vi "file list -- accumulate V2.vi"(11 "file path":path=path "/snowfall/Users/arcadi/Desktop/Ultrasound/Experiment/YBCO_4/Round1/Sweep12/June_2011/062511/221.16400K_300_3100_001_062511.dat") -> (0 "timestamp":dbl[](array[numeric]), 2 "sweep file name array":T1[](array[typedef]), 3 "temperatures":dbl[](array[numeric]))   [LabVIEW 2010]
uses:
  sweep file name.ctl
  <vilib>/Utility/file.llb/Read From Spreadsheet File (string).vi
panel:
  in  "dummy 2":T1={"temperature"=0.0, "temperature str"="", "file path"=path "/snowfall/Users/arcadi/Desktop/Ultrasound/Experiment/YBCO_4/Round1/Sweep12/June_2011/062511/221.16400K_300_3100_001_062511.dat", "last mod"=timestamp(0 s since 1904-01-01), "file name str"="", "mod time(min)"=0.0, "file format"=enum.""}
  in  "sweep file name":T1={"temperature"=0.0, "temperature str"="", "file path"=path "/snowfall/Users/arcadi/Desktop/Ultrasound/Experiment/YBCO_4/Round1/Sweep12/June_2011/062511/221.16400K_300_3100_001_062511.dat", "last mod"=timestamp(0 s since 1904-01-01), "file name str"="", "mod time(min)"=0.0, "file format"=enum.""}
  in  "dummy":T1={"temperature"=0.0, "temperature str"="", "file path"=path "/snowfall/Users/arcadi/Desktop/Ultrasound/Experiment/YBCO_4/Round1/Sweep12/June_2011/062511/221.16400K_300_3100_001_062511.dat", "last mod"=timestamp(0 s since 1904-01-01), "file name str"="", "mod time(min)"=0.0, "file format"=enum.""}
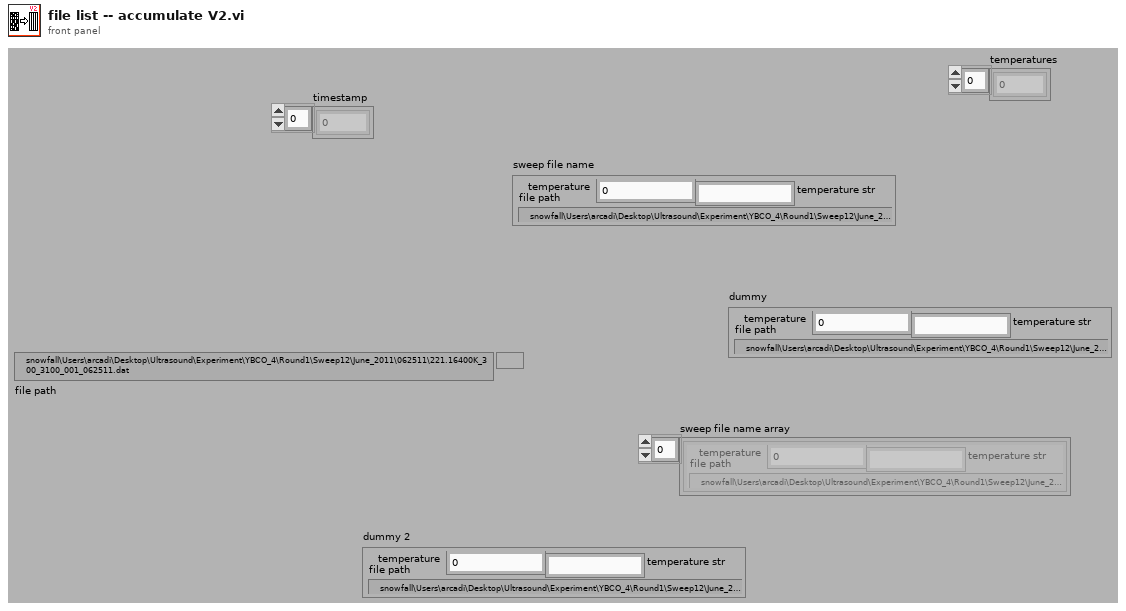
[diagram p1: front panel]
types:
  T1 = typedef "sweep file name.ctl" = cluster{"temperature":dbl, "temperature str":string, "file path":path, "last mod":timestamp, "file name str":string, "mod time(min)":dbl, "file format":enum16{"", "ascii", "binary"}}
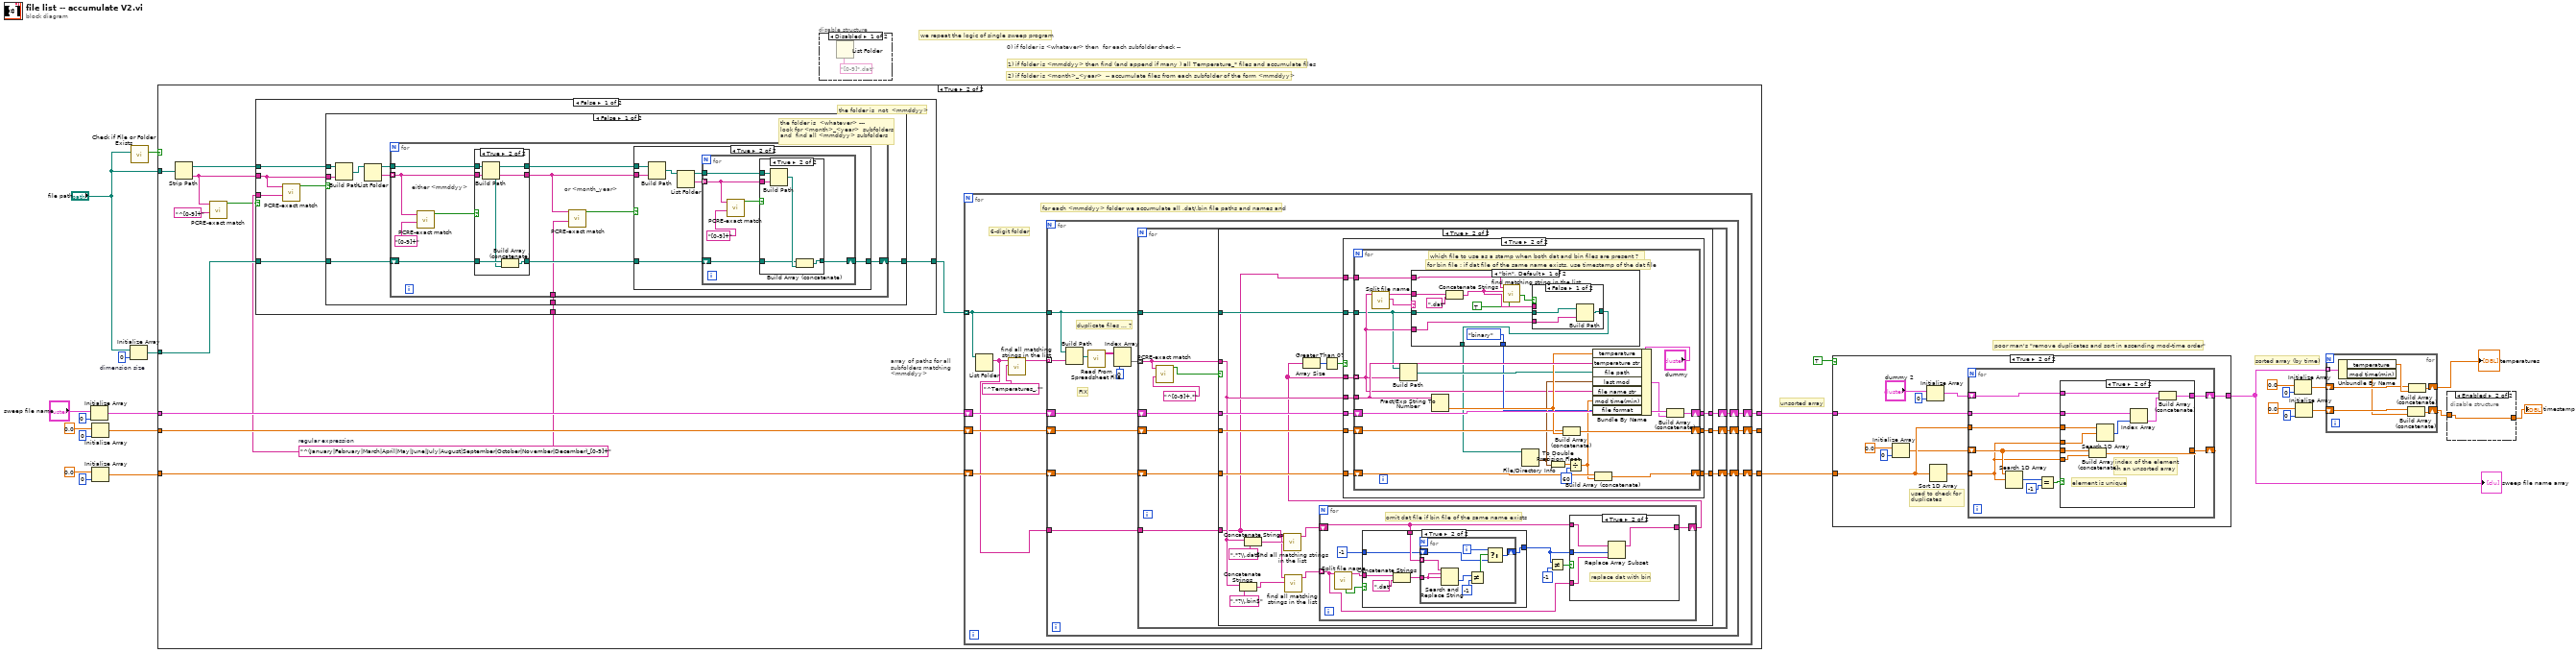
[diagram p0: block diagram]
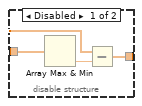
[diagram p2: hidden frame]
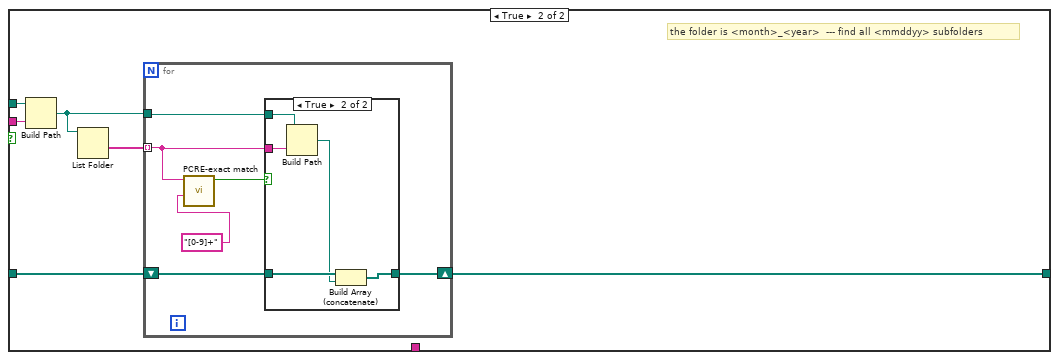
[diagram p10: hidden frame]
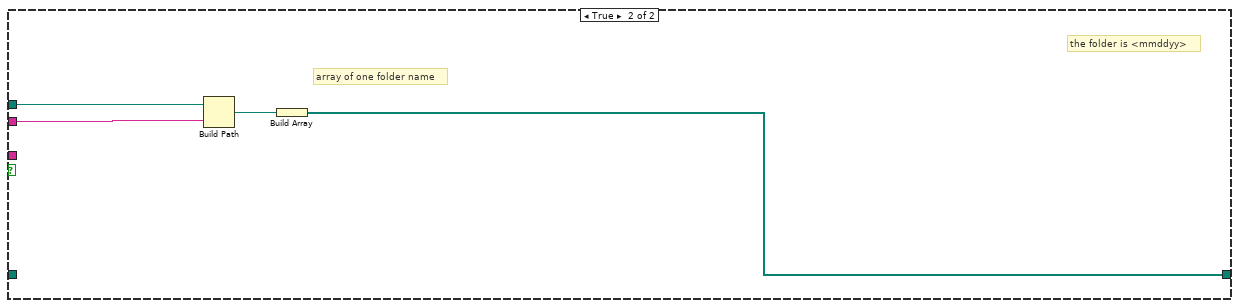
[diagram p12: hidden frame]
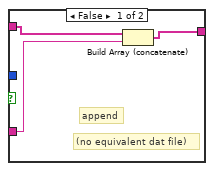
[diagram p14: hidden frame]
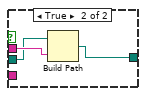
[diagram p17: hidden frame]
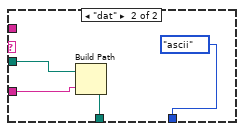
[diagram p18: hidden frame]
diagram:
  w3 = 0  # dimension size
  # "0) if folder is <whatever> then  for each subfolder check --"
  # "sorted array (by time)"
  # "unsorted array"
  # "poor man's \"remove duplicates and sort in ascending mod-time order\""
  # "1) if folder is <mmddyy> then find (and append if many ) all Temperature_* files and accumulate files"
  # "2) if folder is <month>_<year>  -- accumulate files from each subfolder of the form <mmddyy>"
  # "we repeat the logic of single sweep program"
  n1 = Initialize Array("sweep file name", 0 ("dimension size")) -> (w21:T1[])
  n2 = Initialize Array(0.0 ("dimension size"), 0 ("dimension size")) -> (w20:dbl[])
  n3 = Initialize Array(0.0 ("dimension size"), 0 ("dimension size")) -> (w17:dbl[])
  n4 = Initialize Array("file path", w3) -> (w1:path[])
  n5 = call <vilib>:"Check if File or Folder Exists.vi"("path"="file path") -> ("file or folder exists?"=w26:bool)  [unwired: 8 in, 2 out]
  n6 = case shown="True" w26 {
    tunnel: "file path" -> [_ w39]
    tunnel: [w29 w41] -> w14
    tunnel: [w28 w40] -> _
    tunnel: w21 -> [w29 w43]
    tunnel: w20 -> [w28 w42]
    tunnel: w17 -> [w27 w38]
    tunnel: [w27 w37] -> w15
    tunnel: w1 -> [_ w34]
    frame False {
    }
    frame True {
      w33 = "^(January|February|March|April|May|June|July|August|September|October|November|December)_[0-9]+"  # regular expression
      # "array of paths for all  \nsubfolders matching\n<mmddyy>"
      n7 = Strip Path(path=w39) -> (stripped path=w36:path, name=w32:string)
      n8 = call "PCRE-exact match.vi"("regular expression"="^[0-9]+", "input string"=w32) -> ("exact match"=w30:bool)  [unwired: 8 in, 1 out]
      n9 = case shown="False" w30 {
        tunnel: [w50 w118] -> w35
        tunnel: w36 -> [w49 w117]
        tunnel: w32 -> [w45 w116]
        tunnel: w33 -> [w46 _]
        tunnel: w34 -> [w48 _]
        tunnel: w33 -> [w47 _]
        frame False {
          # "the folder is  not  <mmddyy>"
          n10 = call "PCRE-exact match.vi"("regular expression"=w46, "input string"=w45) -> ("exact match"=w44:bool)  [unwired: 8 in, 1 out]
          n11 = case shown="False" w44 {
            tunnel: [w52 w101] -> w50
            tunnel: w45 -> [w55 w100]
            tunnel: w49 -> [w56 w99]
            tunnel: w48 -> [w54 w98]
            tunnel: w47 -> [w53 _]
            frame False {
              # "the folder is  <whatever> --- \nlook for <month>_<year>  subfolders \nand  find all <mmddyy> subfolders"
              n12 = Build Path(base path=w56, name or relative path=w55) -> (appended path=w57:path)
              n13 = List Folder(path=w57) -> (path out=w51:path, folder names=w58:string[])  [unwired: 3 in, 2 out]
              n14 = for {
                tunnel: w58 -> [w64] mode=indexing
                shift-right: [w68] -> w52
                shift-left: w54 -> [w69]
                tunnel: w51 -> [w66]
                tunnel: w53 -> [w60]
                # "or <month_year>"
                # "either <mmddyy>"
                n15 = call "PCRE-exact match.vi"("regular expression"="[0-9]+", "input string"=w64) -> ("exact match"=w62:bool)  [unwired: 8 in, 1 out]
                n16 = case shown="True" w62 {
                  tunnel: w66 -> [w90 w93]
                  tunnel: w64 -> [w91 w94]
                  tunnel: w69 -> [w92 w97]
                  tunnel: [w92 w95] -> w67
                  tunnel: [w91 w94] -> w61
                  tunnel: [w90 w93] -> w65
                  frame False {
                  }
                  frame True {
                    n17 = Build Path(base path=w93, name or relative path=w94) -> (appended path=w96:path)
                    n18 = Build Array (concatenate)(w97, w96) -> (w95:path[])
                  }
                }
                n19 = call "PCRE-exact match.vi"("regular expression"=w60, "input string"=w61) -> ("exact match"=w59:bool)  [unwired: 8 in, 1 out]
                n20 = case shown="True" w59 {
                  tunnel: [w70 w73] -> w68
                  tunnel: w67 -> [w70 w74]
                  tunnel: w65 -> [_ w77]
                  tunnel: w61 -> [_ w76]
                  frame False {
                  }
                  frame True {
                    n21 = Build Path(base path=w77, name or relative path=w76) -> (appended path=w72:path)
                    n22 = List Folder(path=w72) -> (path out=w71:path, folder names=w75:string[])  [unwired: 3 in, 2 out]
                    n23 = for {
                      tunnel: w75 -> [w80] mode=indexing
                      shift-right: [w82] -> w73
                      shift-left: w74 -> [w83]
                      tunnel: w71 -> [w81]
                      n24 = call "PCRE-exact match.vi"("regular expression"="[0-9]+", "input string"=w80) -> ("exact match"=w78:bool)  [unwired: 8 in, 1 out]
                      n25 = case shown="True" w78 {
                        tunnel: w83 -> [w84 w88]
                        tunnel: [w84 w87] -> w82
                        tunnel: w81 -> [_ w86]
                        tunnel: w80 -> [_ w85]
                        frame False {
                        }
                        frame True {
                          n26 = Build Path(base path=w86, name or relative path=w85) -> (appended path=w89:path)
                          n27 = Build Array (concatenate)(w88, w89) -> (w87:path[])
                        }
                      }
                    }
                  }
                }
              }
            }
            frame True {
              # "the folder is <month>_<year>  --- find all <mmddyy> subfolders"
              n28 = Build Path(base path=w99, name or relative path=w100) -> (appended path=w102:path)
              n29 = List Folder(path=w102) -> (folder names=w103:string[])  [unwired: 3 in, 3 out]
              n30 = for {
                tunnel: w103 -> [w106] mode=indexing
                shift-right: [w107] -> w101
                shift-left: w98 -> [w108]
                tunnel: w102 -> [w109]
                n31 = call "PCRE-exact match.vi"("regular expression"="[0-9]+", "input string"=w106) -> ("exact match"=w104:bool)  [unwired: 8 in, 1 out]
                n32 = case shown="True" w104 {
                  tunnel: w109 -> [_ w115]
                  tunnel: w106 -> [_ w114]
                  tunnel: w108 -> [w110 w113]
                  tunnel: [w110 w111] -> w107
                  frame False {
                  }
                  frame True {
                    n33 = Build Path(base path=w115, name or relative path=w114) -> (appended path=w112:path)
                    n34 = Build Array (concatenate)(w113, w112) -> (w111:path[])
                  }
                }
              }
            }
          }
        }
        frame True {
          # "the folder is <mmddyy>"
          # "array of one folder name"
          n35 = Build Path(base path=w117, name or relative path=w116) -> (appended path=w119:path)
          n36 = Build Array(w119) -> (w118:path[])
        }
      }
      n37 = for {
        tunnel: w35 -> [w123] mode=indexing
        shift-right: [w127] -> w41
        shift-left: w43 -> [w129]
        shift-right: [w128] -> w40
        shift-left: w42 -> [w126]
        shift-right: [w124] -> w37
        shift-left: w38 -> [w125]
        # "6-digit folder"
        # "for each <mmddyy> folder we accumulate all .dat/.bin file paths and names and"
        n38 = List Folder(path=w123) -> (filenames=w120:string[])  [unwired: 3 in, 3 out]
        n39 = call "find all matching strings in the list.vi"("regular expression"="^Temperatures_.*" ("pattern"), "strings"=w120) -> ("list of matching strings"=w121:string[])  [unwired: 7 in, 2 out]
        n40 = for {
          tunnel: w121 -> [w133] mode=indexing
          tunnel: w123 -> [w141]
          shift-right: [w135] -> w127
          shift-left: w129 -> [w142]
          shift-right: [w140] -> w128
          shift-left: w126 -> [w134]
          shift-right: [w131] -> w124
          shift-left: w125 -> [w132]
          tunnel: w120 -> [w130]
          # "FIX"
          # "duplicate files ... ?"
          n41 = Build Path(base path=w141, name or relative path=w133) -> (appended path=w139:path)
          n42 = call-poly <vilib>:"Read From Spreadsheet File.vi"("file path (dialog if empty)"=w139) -> ("all rows"=w138:string[][])  [unwired: 6 in, 4 out]
          n43 = Index Array(array=w138, index (col)=0 ("disabled index (col)")) -> (element=w136:string[])  [unwired: 1 in]
          n44 = for {
            tunnel: w136 -> [w146] mode=indexing
            tunnel: w141 -> [w153]
            shift-right: [w151] -> w135
            shift-left: w142 -> [w152]
            shift-right: [w149] -> w140
            shift-left: w134 -> [w150]
            shift-right: [w147] -> w131
            shift-left: w132 -> [w148]
            tunnel: w130 -> [w143]
            n45 = call "PCRE-exact match.vi"("regular expression"="^[0-9]+.*" ("pattern"), "input string"=w146) -> ("exact match"=w145:bool)  [unwired: 8 in, 1 out]
            n46 = case shown="True" w145 {
              tunnel: w153 -> [_ w163]
              tunnel: w146 -> [_ w164]
              tunnel: w152 -> [w155 w173]
              tunnel: [w155 w172] -> w151
              tunnel: w150 -> [w156 w171]
              tunnel: [w156 w170] -> w149
              tunnel: w148 -> [w154 w169]
              tunnel: [w154 w168] -> w147
              tunnel: w143 -> [_ w157]
              frame False {
              }
              frame True {
                n47 = Concatenate Strings(w164, ".*?\\.bin$" ("string")) -> (w160:string)
                n48 = Concatenate Strings(w164, ".*?\\.dat$" ("string")) -> (w161:string)
                n49 = call "find all matching strings in the list.vi"("regular expression"=w161, "strings"=w157) -> ("list of matching strings"=w159:string[])  [unwired: 7 in, 2 out]
                n50 = call "find all matching strings in the list.vi"("regular expression"=w160, "strings"=w157) -> ("list of matching strings"=w158:string[])  [unwired: 7 in, 2 out]
                n51 = for {
                  shift-right: [w177] -> w162
                  shift-left: w159 -> [w178]
                  tunnel: w158 -> [w176] mode=indexing
                  # "omit dat file if bin file of the same name exists"
                  n52 = call "Split file name.vi"("file name"=w176) -> ("name"=w182:string, "exact match"=w183:bool)  [unwired: 8 in, 1 out]
                  n53 = case shown="True" w183 {
                    tunnel: w182 -> [_ w196]
                    tunnel: w178 -> [_ w195]
                    tunnel: [w191 w193] -> w175
                    tunnel: -1 -> [w191 w192]
                    frame False {
                    }
                    frame True {
                      n54 = Concatenate Strings(w196, ".dat" ("string")) -> (w194:string)
                      n55 = for {
                        tunnel: w195 -> [w205] mode=indexing
                        tunnel: w194 -> [w204]
                        shift-right: [w198] -> w193
                        shift-left: w192 -> [w199]
                        i -> [w200]
                        n56 = Search and Replace String(input string=w205, search string=w204, replace string=w204) -> (offset past replacement=w202:i32)  [unwired: 5 in, 3 out]
                        n57 = Not Equal?(x=w202, y=-1) -> (x != y?=w203:bool)
                        n58 = Select(t=w200, s=w203, f=w199) -> (s? t:f=w198:i32)
                      }
                    }
                  }
                  n59 = Not Equal?(x=w175, y=-1) -> (x != y?=w179:bool)
                  n60 = case shown="True" w179 {
                    tunnel: w178 -> [w186 w190]
                    tunnel: [w185 w187] -> w177
                    tunnel: w176 -> [w184 w189]
                    tunnel: w175 -> [_ w188]
                    frame False {
                      # "(no equivalent dat file)"
                      # "append"
                      n61 = Build Array (concatenate)(w186, w184) -> (w185:string[])
                    }
                    frame True {
                      # "replace dat with bin"
                      n62 = Replace Array Subset(array=w190, new element=w189, index=w188) -> (w187:string[])
                    }
                  }
                }
                n63 = Array Size(array=w162) -> (size(s)=w167:i32)
                n64 = Greater Than 0?(x=w167) -> (x > 0?=w166:bool)
                n65 = case shown="True" w166 {
                  tunnel: w162 -> [_ w218]
                  tunnel: w163 -> [_ w217]
                  tunnel: w164 -> [_ w216]
                  tunnel: w173 -> [w208 w215]
                  tunnel: [w208 w212] -> w172
                  tunnel: w171 -> [w207 w214]
                  tunnel: [w207 w211] -> w170
                  tunnel: w169 -> [w206 w213]
                  tunnel: [w206 w210] -> w168
                  tunnel: w157 -> [_ w209]
                  frame False {
                    # "duplicat tempearture folder"
                  }
                  frame True {
                    n66 = for {
                      tunnel: w218 -> [w223] mode=indexing
                      tunnel: w217 -> [w222]
                      tunnel: w216 -> [w239]
                      shift-right: [w231] -> w212
                      shift-left: w215 -> [w238]
                      shift-right: [w230] -> w211
                      shift-left: w214 -> [w235]
                      shift-right: [w229] -> w210
                      shift-left: w213 -> [w233]
                      tunnel: w209 -> [w219]
                      # "which file to use as a stamp when both dat and bin files are present ?"
                      # "for bin file : if dat file of the same name exists, use timestamp of the dat file"
                      n67 = call "Split file name.vi"("file name"=w223) -> ("extension"=w224:string, "name"=w220:string)  [unwired: 8 in, 1 out]
                      n68 = Build Path(base path=w222, name or relative path=w223) -> (appended path=w234:path)
                      n69 = case shown="\"bin\", Default" w224 {
                        tunnel: [enum16{"", "ascii", "binary"}."binary" ("action") enum16{"", "ascii", "binary"}."ascii" ("action")] -> w225
                        tunnel: w223 -> [w246 w259]
                        tunnel: w222 -> [w245 w258]
                        tunnel: [w247 w257] -> w221
                        tunnel: w220 -> [w248 _]
                        tunnel: w219 -> [w244 _]
                        frame "bin", Default {
                          n70 = Concatenate Strings(w248, ".dat" ("string")) -> (w242:string)
                          n71 = call "find matching string in the list.vi"("quote specials"=TRUE, "regular expression"=w242, "strings"=w244) -> ("match found"=w243:bool)  [unwired: 6 in, 2 out]
                          n72 = case shown="False" w243 {
                            tunnel: [w251 w254] -> w247
                            tunnel: w245 -> [w253 w255]
                            tunnel: w246 -> [w252 _]
                            tunnel: w242 -> [_ w256]
                            frame False {
                              n73 = Build Path(base path=w253, name or relative path=w252) -> (appended path=w251:path)
                            }
                            frame True {
                              n74 = Build Path(base path=w255, name or relative path=w256) -> (appended path=w254:path)
                            }
                          }
                        }
                        frame "dat" {
                          n75 = Build Path(base path=w258, name or relative path=w259) -> (appended path=w257:path)
                        }
                      }
                      n76 = Fract/Exp String To Number(string=w239) -> (number=w236:dbl)  [unwired: 3 in, 1 out]
                      n77 = File/Directory Info(path=w221) -> (last mod=w232:timestamp)  [unwired: 1 in, 6 out]
                      n78 = To Double Precision Float(number=w232) -> (double precision float=w228:dbl)
                      n79 = Build Array (concatenate)(w235, w236) -> (w230:dbl[])
                      n80 = Divide(x=w228, y=60) -> (x/y=w226:dbl)
                      n81 = Bundle By Name(cluster="dummy", "temperature"=w236, "temperature str"=w239, "file path"=w234, "last mod"=w232, "file name str"=w223, "mod time(min)"=w226, "file format"=w225) -> (w237:T1)
                      n82 = Build Array (concatenate)(w233, w226) -> (w229:dbl[])
                      n83 = Build Array (concatenate)(w238, w237) -> (w231:T1[])
                    }
                  }
                }
              }
            }
          }
        }
      }
    }
  }
  n84 = disable-structure shown="Disabled" {
    frame Disabled {
      n85 = List Folder(pattern="[0-9]*.dat") -> ()  [unwired: 3 in, 4 out]
    }
    frame Enabled {
    }
  }
  n86 = case shown="True" TRUE {
    tunnel: w15 -> [_ w266]
    tunnel: w14 -> [w262 w271]
    tunnel: [w262 w270] -> w4
    frame False {
    }
    frame True {
      # "used to check for \nduplicates"
      n87 = Initialize Array(0.0 ("dimension size"), 0 ("dimension size")) -> (w263:dbl[])
      n88 = Initialize Array("dummy 2", 0 ("dimension size")) -> (w267:T1[])
      n89 = Sort 1D Array(array=w266) -> (sorted array=w272:dbl[])
      n90 = for {
        shift-right: [w279] -> w270
        shift-left: w267 -> [w278]
        shift-right: [w277] -> _
        shift-left: w263 -> [w276]
        tunnel: w272 -> [w273] mode=indexing
        tunnel: w266 -> [w275]
        tunnel: w271 -> [w274]
        n91 = Search 1D Array(1D array=w276, element=w273) -> (index of element=w282:i32)  [unwired: 1 in]
        n92 = Equal?(x=w282, y=-1) -> (x = y?=w280:bool)
        n93 = case shown="True" w280 {
          tunnel: [w284 w293] -> w279
          tunnel: w278 -> [w284 w294]
          tunnel: [w283 w285] -> w277
          tunnel: w276 -> [w283 w287]
          tunnel: w275 -> [_ w292]
          tunnel: w273 -> [_ w291]
          tunnel: w274 -> [_ w289]
          tunnel: w273 -> [_ w286]
          frame False {
            # "element is not unique"
          }
          frame True {
            # "index of the element \nin an unsorted array"
            # "element is unique"
            n94 = Build Array (concatenate)(w287, w286) -> (w285:dbl[])
            n95 = Search 1D Array(1D array=w292, element=w291) -> (index of element=w290:i32)  [unwired: 1 in]
            n96 = Index Array(array=w289, index=w290) -> (element=w288:T1)
            n97 = Build Array (concatenate)(w294, w288) -> (w293:T1[])
          }
        }
      }
    }
  }
  "sweep file name array" <- w4
  n98 = Initialize Array(0.0 ("dimension size"), 0 ("dimension size")) -> (w11:dbl[])
  n99 = Initialize Array(0.0 ("dimension size"), 0 ("dimension size")) -> (w8:dbl[])
  n100 = for {
    tunnel: w4 -> [w301] mode=indexing
    shift-right: [w295] -> w7
    shift-left: w11 -> [w299]
    shift-right: [w296] -> w6
    shift-left: w8 -> [w298]
    n101 = Unbundle By Name(w301) -> ("temperature"=w300:dbl, "mod time(min)"=w297:dbl)
    n102 = Build Array (concatenate)(w298, w297) -> (w296:dbl[])
    n103 = Build Array (concatenate)(w299, w300) -> (w295:dbl[])
  }
  "temperatures" <- w7
  n104 = disable-structure shown="Enabled" {
    disable-tunnel: w6 -> [w303 w305]
    disable-tunnel: [w302 w305] -> w5
    frame Disabled {
      n105 = Array Max & Min(array=w303) -> (min value=w304:dbl)  [unwired: 3 out]
      n106 = Subtract(x=w303, y=w304) -> (x-y=w302:dbl[])
    }
    frame Enabled {
    }
  }
  "timestamp" <- w5
